vi "st_Percentiles (array).vi"(10 "p array":dbl[](array[numeric]), 11 "x array":dbl[](array[numeric])) -> (0 "error":i32, 3 "percentiles":dbl[](array[numeric]))   [LabVIEW 2020, in "NI_Gmath.lvlib"]
doc: "Computes a value that is greater than <B>p</B> percent of the data values in <B>x array</B>. Wire data to the <B>p</B> input to determine the polymorphic instance to use or manually select the instance."
uses:
  <vilib>/gmath/NI_Gmath.lvlib
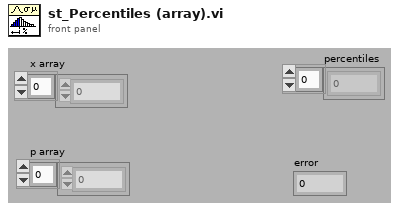
[diagram p1: front panel]
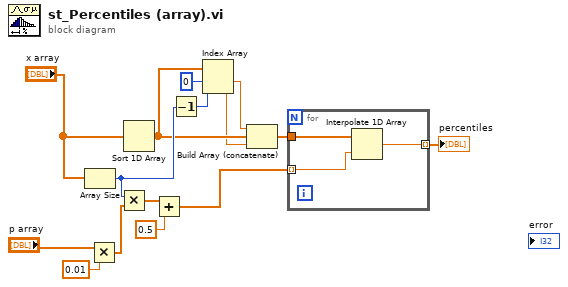
[diagram p0: block diagram]
diagram:
  n1 = Array Size(array="x array") -> (size(s)=w8:i32)
  n2 = Multiply(x="p array", y=0.01) -> (x*y=w13:dbl[])
  n3 = Multiply(x=w8, y=w13) -> (x*y=w12:dbl[])
  n4 = Sort 1D Array(array="x array") -> (sorted array=w6:dbl[])
  n5 = Add(x=w12, y=0.5) -> (x+y=w1:dbl[])
  n6 = Decrement(x=w8) -> (x-1=w9:i32)
  n7 = Index Array(array=w6, index #1=0 ("index"), index #2=w9) -> (element #1=w7:dbl, element #2=w5:dbl)
  n8 = Build Array (concatenate)(w7, w6, w5) -> (w4:dbl[])
  n9 = for {
    tunnel: w4 -> [w18]
    tunnel: [w17] -> w3 mode=indexing
    tunnel: w1 -> [w16] mode=indexing
    n10 = Interpolate 1D Array(1:w16, 2:w18) -> (0:w17:dbl)
  }
  "percentiles" <- w3
